vi "Drive Controller.vi"(8 "error in":errorcluster) -> ()   [LabVIEW 2017]
doc: "This VI executes continuously carrying out the current operation and responding to updates or new operation requests. It will often contain the timing or control code that is difficult to place directly in TeleOp. This VI generally opens all sensors and motors and isolates the rest of the robot code from knowing implementation details of how the operations are carried out."
uses:
  Drive Operations.ctl
  Drive Setpoints.ctl
  <vilib>/Rock Robotics/WPI/SafetyOutput/WPI_SafetyOutputConfigMenu.ctl
  <vilib>/Rock Robotics/WPI/RobotDrive/WPI_RobotDriveOpen2MotorWithTalon.vi
  <vilib>/Rock Robotics/SystemInterfaces/DIO/FPGA_DIOPWMChannel.ctl
  <vilib>/Rock Robotics/WPI/Gyro/WPI_GyroXRS450_SPI_Open.vi
  <vilib>/Rock Robotics/WPI/Framework/Completion Status.ctl
  <vilib>/Rock Robotics/SystemInterfaces/spilib/spi_bus.ctl
panel:
  in  "SPI Bus":T1
  in  "Sample Rate (Hz)":dbl=1000.0 min=50.0 max=20000.0 format="%#_13g"
  in  "Interactive Values":T2
  in  "Buttons":cluster{"Execute Cmd":bool, "Abort Cmd":bool}
  out "Command Timing":cluster{"Start Time (ms)":u32, "Iterations":i32}
  out "Status":T4
  out "Setpoints":T5(graph)
  out "Current\nCmd":string
  # "Tip: The graph shows the motor setpoints. It may also be helpful to observe inputs and sensor values.\nYou may also want to display tuning or debugging controls."
  # "Interactive Command: You may fill in the settings for a command\nand schedule it with the Execute button. You can observe and abort\nany command while fine tuning the code for the controller."
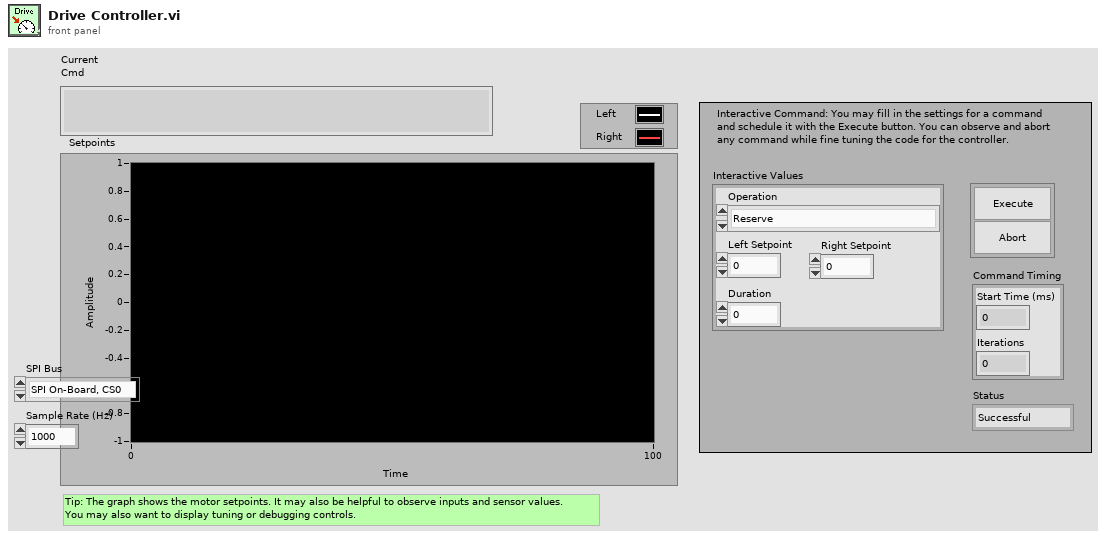
[diagram p1: front panel]
types:
  T1 = typedef "spi_bus.ctl" = enum16{"SPI On-Board, CS0", "SPI On-Board, CS1", "SPI On-Board, CS2", "SPI On-Board, CS3", "SPI MXP", "Invalid"}
  T2 = typedef "Drive Setpoints.ctl" = cluster{"Operation":T3, "Left Setpoint":dbl, "Right Setpoint":dbl, "Duration":dbl}
  T3 = typedef "Drive Operations.ctl" = enum16{"Reserve", "Read Current", "Freestyle", "Drive for Distance", "Turn Angle", "Guided Drive"}
  T4 = typedef "Completion Status.ctl" = enum16{"Successful", "Aborted", "Incomplete"}
  T5 = cluster{"Left Setpoint":dbl, "Right Setpoint":dbl}
  T6 = typedef "FPGA_DIOPWMChannel.ctl" = enum8{"PWM 0", "PWM 1", "PWM 2", "PWM 3", "PWM 4", "PWM 5", "PWM 6", "PWM 7", "PWM 8", "PWM 9", "PWM MXP 0", "PWM MXP 1", "PWM MXP 2", "PWM MXP 3", "PWM MXP 4", "PWM MXP 5", "PWM MXP 6", "PWM MXP 7", "PWM MXP 8", "PWM MXP 9", "Invalid"}
  T7 = typedef "WPI_SafetyOutputConfigMenu.ctl" = enum16{"Enable", "Disable"}
  T8 = typedef "WPI_GyroDevRef.ctl" = cluster{"DevStatus":errorcluster, "Analog Channel":T9, "Gain (VoltsPerDegree/Second)":dbl, "Gyro Type":enum16{"Analog", "XRS450"}, "Handle":i32, "SPI Bus":T1, "Device Found":bool, "Sample Rate":dbl, "Calibrate On Open":bool, "Offset":dbl}
  T9 = typedef "FPGA_AIChannel.ctl" = enum8{"AI 0", "AI 1", "AI 2", "AI 3", "AI MXP 0", "AI MXP 1", "AI MXP 2", "AI MXP 3", "Invalid"}
  T10 = typedef "WPI_RobotDriveDevRef.ctl" = cluster{"DevStatus":errorcluster, "Motors[]":T11[], "Square Inputs":bool, "Max Output":dbl}
  T11 = typedef "WPI_MotorControlDeviceRef.ctl" = cluster{"DeviceStatus":errorcluster, "Type":T12, "PWM":cluster{"PWM Channel":T6, "DeadBand":T13}, "CAN":cluster{"Device Number":u8, "SetOutput VI Ref":variant, "GetOutput VI Ref":variant, "Enable VI Ref":variant, "Disable VI Ref":variant, "Data":variant}, "Invert":bool, "DIO PWM":cluster{"PWM \"Enable\" Channel":T6, "DIOChannel":T14, "PWM Rate":dbl}}
  T12 = typedef "WPI_MotorControlType.ctl" = enum16{"PWM", "CAN", "DIO PWM"}
  T13 = typedef "WPI_PWMDeadband.ctl" = cluster{"Name":string, "maxPositivePwm":i32, "minPositivePwm":i32, "centerPwm":i32, "maxNegativePwm":i32, "minNegativePwm":i32, "angularRange":u16}
  T14 = typedef "FPGA_DIOChannel.ctl" = enum8{"DIO 0", "DIO 1", "DIO 2", "DIO 3", "DIO 4", "DIO 5", "DIO 6", "DIO 7", "DIO 8", "DIO 9", "DIO MXP 0", "DIO MXP 1", "DIO MXP 2", "DIO MXP 3", "DIO MXP 4", "DIO MXP 5", "DIO MXP 6", "DIO MXP 7", "DIO MXP 8", "DIO MXP 9", "DIO MXP 10", "DIO MXP 11", "DIO MXP 12", "DIO MXP 13", "DIO MXP 14", "DIO MXP 15", "SPI Port CS1", "SPI Port CS2", "SPI Port CS3", "SPI Port MISO", "SPI Port MOSI", "Invalid"}
  T15 = typedef "Command Status Info.ctl" = cluster{"Name":string, "Status":T4, "notifier out":T16}
  T16 = typedef "Completion Notifier.ctl" = refnum<notifier>
  T17 = cluster{"SubSystem Data":T2, cluster{"Start Time (ms)":u32, "Iterations":i32}, cluster{"Command Info":T15, "Description":string, "Default Command":T2, "queue out":refnum<queue>, "Subsystem Name":string}}
  T18 = cluster{"SubSystem Data":T2, cluster{"Start Time (ms)":u32, "Iterations":i32}, "Default Command Arguments":cluster{"Command Info":T15, "Description":string, "Default Command":T2, "queue out":refnum<queue>, "Subsystem Name":string}}
  T19 = cluster{"Don't move motors while reserved":dbl, "Don't move motors while reserved":dbl}
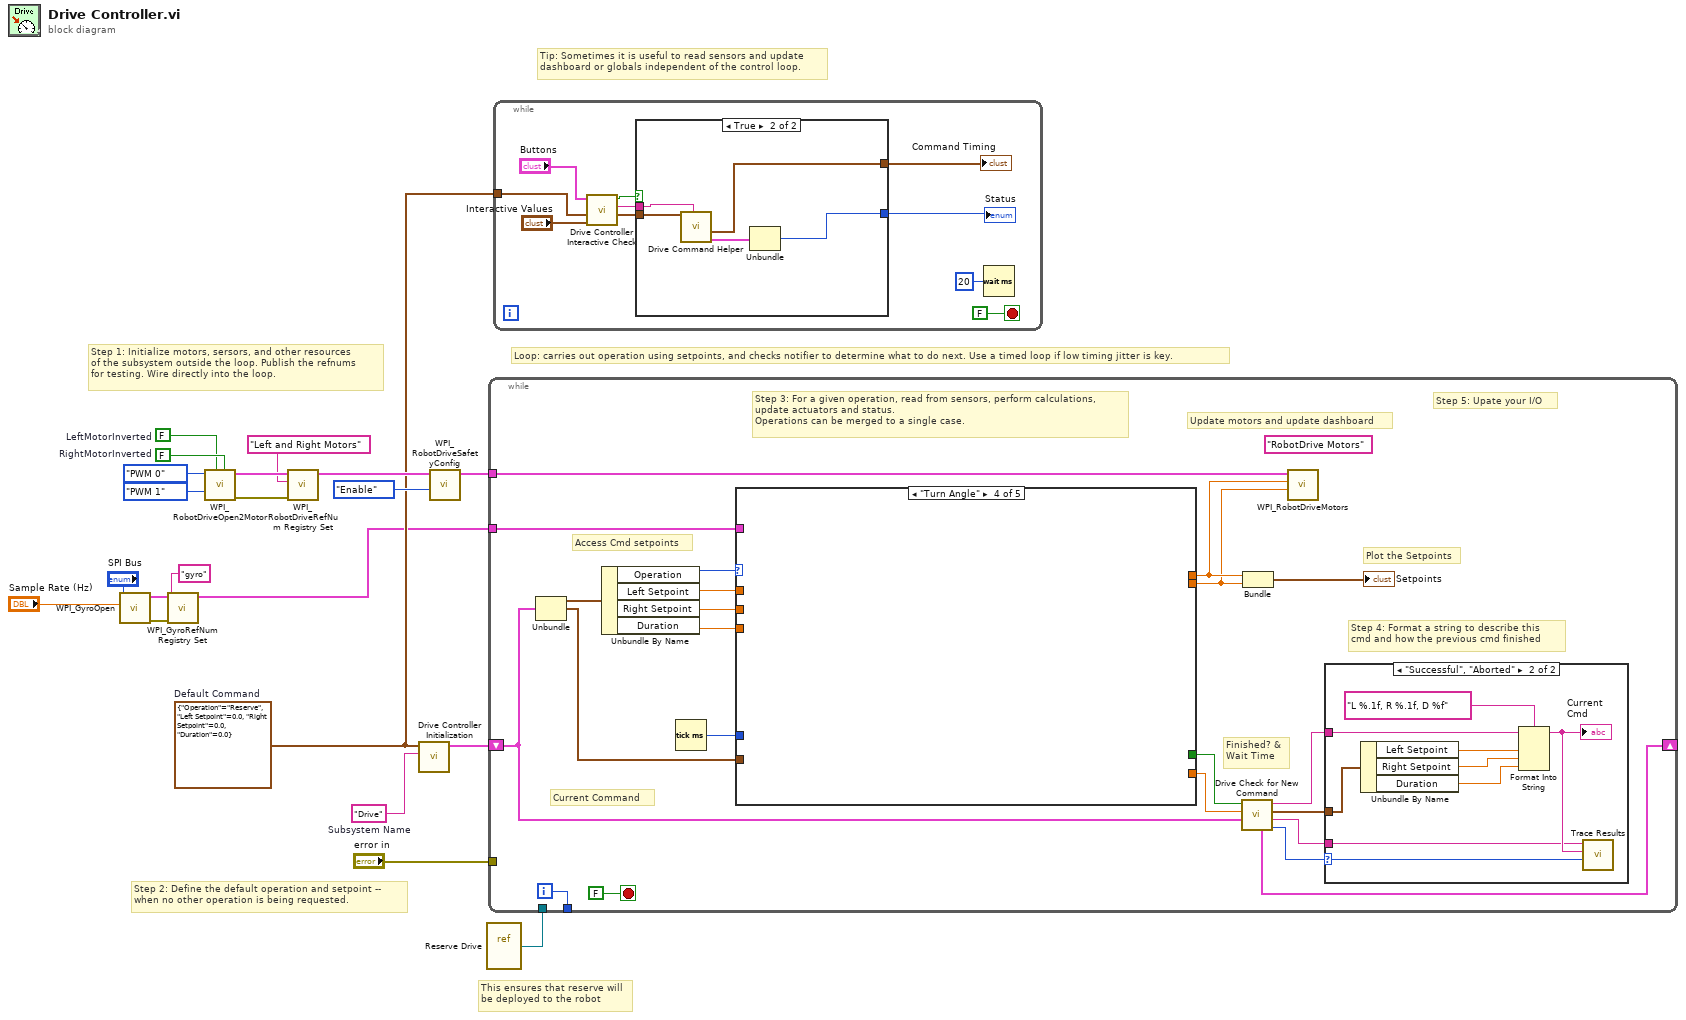
[diagram p0: block diagram]
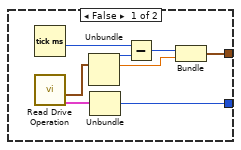
[diagram p2: hidden frame]
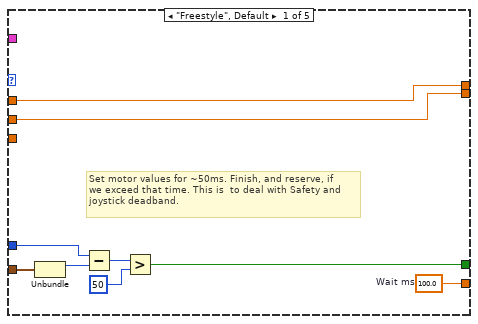
[diagram p4: hidden frame]
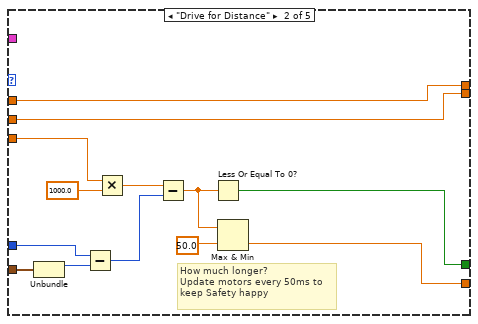
[diagram p5: hidden frame]
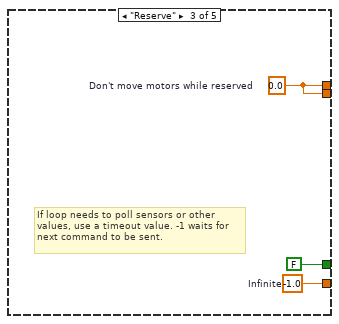
[diagram p6: hidden frame]
diagram:
  w19 = FALSE  # LeftMotorInverted
  w20 = FALSE  # RightMotorInverted
  w9 = T2 {"Operation"=enum."Reserve", "Left Setpoint"=0.0, "Right Setpoint"=0.0, "Duration"=0.0}  # Default Command
  w21 = "Drive"  # Subsystem Name
  # "This ensures that reserve will\nbe deployed to the robot"
  # "Tip: Sometimes it is useful to read sensors and update\ndashboard or globals independent of the control loop."
  # "Step 2: Define the default operation and setpoint --\nwhen no other operation is being requested."
  # "Step 1: Initialize motors, sersors, and other resources\nof the subsystem outside the loop. Publish the refnums\nfor testing. Wire directly into the loop."
  # "Loop: carries out operation using setpoints, and checks notifier to determine what to do next. Use a timed loop if low timing jitter is key."
  n1 = call-poly <vilib>:"WPI_GyroOpen.vi"("Sample Rate (Hz)"="Sample Rate (Hz)", "SPI Bus"="SPI Bus") -> ("error out"=w4:errorcluster, "GyroDevRef"=w3:T8)  [unwired: 7 in, 1 out]
  n2 = call <vilib>:"WPI_GyroRefNum Registry Set.vi"("error in (no error)"=w4, "refnum name"="gyro", "GyroDevRef"=w3) -> ("GyroDevRef"=w1:T8)  [unwired: 7 in, 1 out]
  n3 = call-poly <vilib>:"WPI_RobotDriveOpen2Motor.vi"("Right Motor Inverted"=w20, "Left Motor Inverted"=w19, "Right Motor"=FPGA_DIOPWMChannel."PWM 1", "Left Motor"=FPGA_DIOPWMChannel."PWM 0") -> ("error out"=w16:errorcluster, "RobotDriveDevRef"=w18:T10)  [unwired: 1 in, 5 out]
  n4 = call <vilib>:"WPI_RobotDriveRefNum Registry Set.vi"("error in (no error)"=w16, "refnum name"="Left and Right Motors", "RobotDriveDevRef"=w18) -> ("RobotDriveDevRef"=w15:T10)  [unwired: 1 in, 7 out]
  n5 = call "Drive Controller Initialization.vi"("Subsystem Name"=w21, "Default Command"=w9) -> ("Current Command"=w11:T17)  [unwired: 9 in]
  n6 = call <vilib>:"WPI_RobotDriveSafetyConfig.vi"("mode"=WPI_SafetyOutputConfigMenu."Enable", "RobotDriveDevRef"=w15) -> ("RobotDriveDevRef"=w13:T10)  [unwired: 8 in, 1 out]
  n7 = vi-ref "Reserve Drive.vi"() -> (w10:refnum<vi>)
  n8 = while {
    shift-right: [w30] -> _
    shift-left: w11 -> [w23]
    tunnel: [w42] -> _
    tunnel: w13 -> [w38]
    tunnel: "error in" -> [_]
    tunnel: w10 -> [_]
    tunnel: w1 -> [w22]
    i -> [w42]
    stop <- FALSE stop-if-true
    (unwired) "RobotDrive Motors" ("Name")
    # "Step 5: Upate your I/O"
    # "Step 4: Format a string to describe this\ncmd and how the previous cmd finished"
    # "Current Command"
    # "Update motors and update dashboard"
    # "Plot the Setpoints"
    # "Access Cmd setpoints"
    # "Finished? &\nWait Time"
    # "Step 3: For a given operation, read from sensors, perform calculations,\nupdate actuators and status.\nOperations can be merged to a single case."
    n9 = Unbundle(w23) -> ("SubSystem Data"=w37:T2, w24:cluster{"Start Time (ms)":u32, "Iterations":i32})  [unwired: 1 out]
    n10 = Unbundle By Name(w37) -> ("Operation"=w36:T3, "Left Setpoint"=w35:dbl, "Right Setpoint"=w34:dbl, "Duration"=w33:dbl)
    n11 = Tick Count (ms)() -> (millisecond timer value=w32:u32)
    n12 = case shown="\"Turn Angle\"" w36 {
      tunnel: [w61 w62 w77 _ _] -> w29
      tunnel: [w54 w69 FALSE ("ignore previous (F)") _ _] -> w28
      tunnel: w24 -> [w53 w71 _ _ _]
      tunnel: [w60 w68 w75 _ _] -> w40
      tunnel: [w59 w67 w75 _ _] -> w39
      tunnel: w35 -> [w60 w68 _ _ _]
      tunnel: w34 -> [w59 w67 _ _ _]
      tunnel: w33 -> [_ w66 _ _ _]
      tunnel: w32 -> [w55 w65 _ _ _]
      tunnel: w22 -> [_ _ _ _ _]
      frame "Freestyle", Default {
        w61 = 100.0  # Wait ms
        # "Set motor values for ~50ms. Finish, and reserve, if\nwe exceed that time. This is  to deal with Safety and\njoystick deadband."
        n13 = Unbundle(w53) -> ("Start Time (ms)"=w56:u32)  [unwired: 1 out]
        n14 = Subtract(x=w55, y=w56) -> (x-y=w57:u32)
        n15 = Greater?(x=w57, y=u8 50 ("Left Motor")) -> (0:w54:bool)
      }
      frame "Drive for Distance" {
        # "How much longer?\nUpdate motors every 50ms to\nkeep Safety happy"
        n16 = Unbundle(w71) -> ("Start Time (ms)"=w70:u32)  [unwired: 1 out]
        n17 = Subtract(x=w65, y=w70) -> (x-y=w74:u32)
        n18 = Multiply(x=w66, y=1000.0) -> (x*y=w73:dbl)
        n19 = Subtract(x=w73, y=w74) -> (x-y=w64:dbl)
        n20 = Less Or Equal To 0?(x=w64) -> (x <= 0?=w69:bool)
        n21 = Max & Min(x=w64, y=50.0) -> (min(x,y)=w62:dbl)  [unwired: 1 out]
      }
      frame "Reserve" {
        w75 = 0.0  # Don't move motors while reserved
        w77 = -1.0  # Infinite
        # "If loop needs to poll sensors or other\nvalues, use a timeout value. -1 waits for\nnext command to be sent."
      }
      frame "Turn Angle" {
      }
      frame "Guided Drive" {
      }
    }
    n22 = call "Drive Check for New Command.vi"("input cluster"=w23, "Wait time (ms)"=w29, "Finished?"=w28) -> ("Completion"=w31:T4, "Subsystem Name"=w25:string, "Current Command"=w26:T2, "Initial Trace String"=w27:string, "Next Command"=w30:T18)  [unwired: 4 in]
    n23 = Bundle("Don't move motors while reserved"=w40, "Don't move motors while reserved"=w39) -> (→"Setpoints":T19)  [unwired: 1 in]
    n24 = call <vilib>:"WPI_RobotDriveMotors.vi"("RightSpeed"=w39, "LeftSpeed"=w40, "RobotDriveDevRef"=w38) -> ()  [unwired: 1 in, 8 out]
    n25 = case shown="\"Successful\", \"Aborted\"" w31 {
      selector: w31 -> [_ w52]
      tunnel: w27 -> [_ w47]
      tunnel: w26 -> [_ w48]
      tunnel: w25 -> [_ w44]
      frame "Incomplete", Default {
        # "Continuing current command"
      }
      frame "Successful", "Aborted" {
        # "Report and setup for next command"
        n26 = Unbundle By Name(w48) -> ("Left Setpoint"=w50:dbl, "Right Setpoint"=w51:dbl, "Duration"=w45:dbl)
        n27 = Format Into String(format string="L %.1f, R %.1f, D %f", initial string=w47, w50, w51, w45) -> (resulting string=w46:string)  [unwired: 1 in, 1 out]
        "Current\nCmd" <- w46
        n28 = call <vilib>:"Trace Results.vi"("Status of previous command"=w52, "Description"=w46, "Subsystem"=w44) -> ()  [unwired: 9 in]
      }
    }
  }
  n29 = while {
    tunnel: w9 -> [w79]
    stop <- FALSE stop-if-true
    n30 = call "Drive Controller Interactive Check.vi"("Interactive Command In"="Interactive Values", "Default Command"=w79, "Buttons"="Buttons") -> ("Interactive Command Out"=w81:T2, "Trace String"=w82:string, "Schedule"=w83:bool)  [unwired: 6 in]
    n31 = case shown="True" w83 {
      tunnel: [w92 w100] -> w84
      tunnel: [w91 w96] -> w85
      tunnel: w82 -> [_ w98]
      tunnel: w81 -> [_ w97]
      frame False {
        n32 = Tick Count (ms)() -> (millisecond timer value=w95:u32)
        n33 = call "Read Drive Operation.vi"() -> ("Command Info"=w89:T15, "SubSystem Data"=w88:T2)  [unwired: 9 in, 1 out]
        n34 = Unbundle(w88) -> ("Operation"=w93:T3, "Left Setpoint"=w90:dbl)  [unwired: 2 out]
        n35 = Unbundle(w89) -> ("Status"=w92:T4)  [unwired: 2 out]
        n36 = Subtract(x=w95, y=w93) -> (x-y=w94:u32)
        n37 = Bundle(w94, "Left Setpoint"=w90) -> (w91:cluster{u32, "Left Setpoint":dbl})  [unwired: 1 in]
      }
      frame True {
        n38 = call "Drive Command Helper.vi"("Description"=w98, "SubSystem Data"=w97) -> ("Command Info Out"=w99:T15, "Command Timing"=w96:cluster{"Start Time (ms)":u32, "Iterations":i32})  [unwired: 7 in, 1 out]
        n39 = Unbundle(w99) -> ("Status"=w100:T4)  [unwired: 2 out]
      }
    }
    "Status" <- w84
    "Command Timing" <- w85
    n40 = Wait (ms)(milliseconds to wait=u32 20) -> ()  [unwired: 1 out]
  }
